vi "Update Nested State.vi"(8 "error in (no error)":errorcluster, 9 "State":T1, 10 "Task Hierarchy":T2, 11 "VolatusCore in":refnum<class "VolatusCore.lvclass">) -> (0 "error out":errorcluster, 3 "VolatusCore out":refnum<class "VolatusCore.lvclass">)   [LabVIEW 2020, in "Volatus.lvlib" / "VolatusCore.lvclass"]
uses:
  VolatusCore.lvclass
  Task Hierarchy.ctl
  Task State.ctl
  Volatus.lvlib
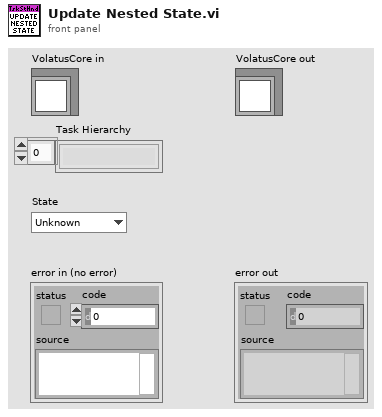
[diagram p1: front panel]
types:
  T1 = typedef "Volatus.lvlib/Task State.ctl" = enum16{"Unknown", "Idle", "Initializing", "Starting", "Running", "Stopping", "Stopped", "Error - Init", "Error - Start", "Error - Run", "Error - Stop"}
  T2 = typedef "Volatus.lvlib/Task Hierarchy.ctl" = string[]
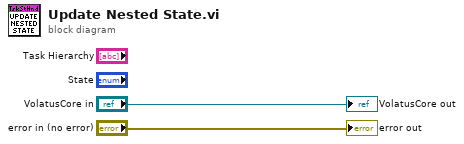
[diagram p0: block diagram]
diagram:
  "error out" <- "error in (no error)"
  "VolatusCore out" <- "VolatusCore in"
